vi "S2C_OM8257_Proc_Close.vi"(8 "Error In":errorcluster) -> (0 "Error Out":errorcluster)   [LabVIEW 2015]
uses:
  S2C_OM8257_Proc_Globals.vi
  <instrlib>/Associated Research 82XX/Associated Research 82XX.lvlib
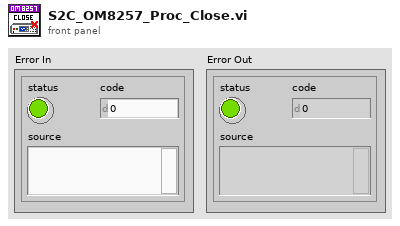
[diagram p1: front panel]
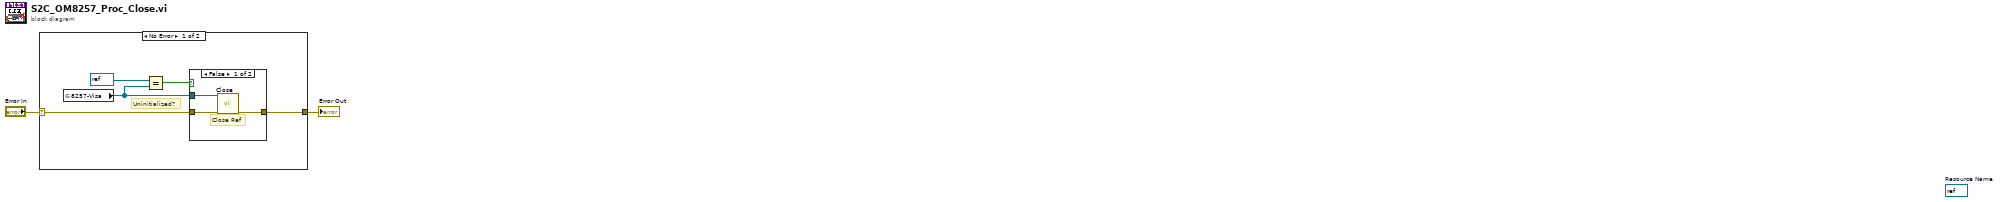
[diagram p0: block diagram]
diagram:
  (unwired) refnum<visa-resource-name> refnum  # Resource Name
  n1 = case shown="No Error" "Error In" {
    selector: "Error In" -> [w7 w12]
    tunnel: [w4 w12] -> w1
    frame No Error {
      # "Uninitialized?"
      n2 = global read "S2C_OM8257_Proc_Globals.vi" "8257-Visa"() -> (w3:refnum<visa-resource-name>)
      n3 = Equal?(x=refnum<visa-resource-name> refnum ("SerialRef"), y=w3) -> (x = y?=w6:bool)
      n4 = case shown="False" w6 {
        tunnel: w7 -> [w10 w11]
        tunnel: [w9 w11] -> w4
        tunnel: w3 -> [w8 _]
        frame False {
          # "Close Ref"
          n5 = call <instrlib>:"Close.vi"("VISA resource name"=w8, "error in (no error)"=w10) -> ("error out"=w9:errorcluster)  [unwired: 13 in]
        }
        frame True {
        }
      }
    }
    frame Error {
    }
  }
  "Error Out" <- w1
